vi "Lifter.vi"(1 "Joystick Speed":dbl=-0.031496062992125984) -> (0 "In Position":bool=TRUE)   [LabVIEW 2013]
uses:
  Robot Global Data.vi
  <vilib>/Rock Robotics/WPI/Joystick/WPI_JoystickGetSetRefNum.vi
panel:
  in  "Adjustment (V)":dbl
  in  "Adjust Gain (V/ms)":dbl=0.01
  in  "Limits":cluster{"Upper":dbl, "Lower":dbl}={"Upper"=3.62, "Lower"=2.5}
  out "Pot Voltage":dbl=3.41879165
  in  "Tolerance":dbl=0.01
  in  "Position Voltages":dbl[](array[numeric])=[2.5, 3.32, 3.48, 0.7, 0.7]
  in  "Motor Gain":dbl=15.0
  # "0 - Climb\n1 - Load\n2 - Pre-climb\n3 - Shoot"
  # "0 - Climb"
  # "2.5"
  # "1 - Load"
  # "3.42"
  # "3.48"
  # "2 - Pre-climb"
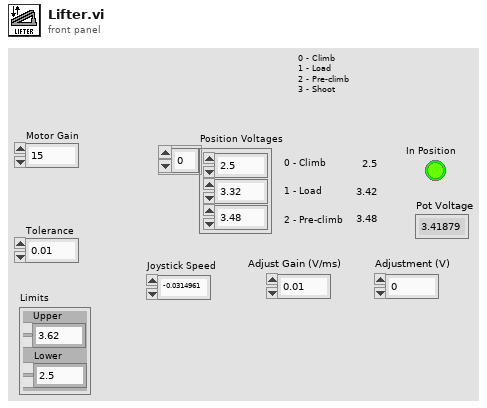
[diagram p1: front panel]
types:
  T1 = typedef "WPI_JoystickDevRef.ctl" = cluster{"Device":T2}
  T2 = typedef "WPI_JoystickDeviceEnum.ctl" = enum16{"USB 1", "USB 2", "USB 3", "USB 4", "Kinect 1", "Kinect 2"}
  T3 = typedef "WPI_AnalogChannelDevRef.ctl" = cluster{"DevStatus":errorcluster, "Analog Module":T4, "Analog Channel":T5}
  T4 = typedef "FPGA_TypedefAnalogModule.ctl" = enum16{"Analog Module 1", "Analog Module 2"}
  T5 = typedef "FPGA_AIChannel.ctl" = enum8{"AI 1", "AI 2", "AI 3", "AI 4", "AI 5", "AI 6", "AI 7", "AI 8", "Invalid"}
  T6 = typedef "WPI_JoystickButtonState.ctl" = cluster{"Button 1":bool, "Button 2":bool, "Button 3":bool, "Button 4":bool, "Button 5":bool, "Button 6":bool, "Button 7":bool, "Button 8":bool, "Button 9":bool, "Button 10":bool, "Button 11":bool, "Button 12":bool}
  T7 = typedef "WPI_MotorControlDeviceRef.ctl" = cluster{"DeviceStatus":errorcluster, "Type":enum16{"PWM", "CAN"}, "PWM":cluster{"Digital Module":T8, "PWM Channel":T9, "DeadBand":T10}, "CAN":cluster{"Device Number":u8, "Control Mode":T11, "Semaphore":T12, "Max Vout":dbl}, "Invert":bool, "TransformRef":T13, "InvTransformRef":T13}
  T8 = typedef "FPGA_TypedefDigitalModule.ctl" = enum16{"Digital Module 1", "Digital Module 2"}
  T9 = typedef "FPGA_DIOPWMChannel.ctl" = enum8{"PWM 1", "PWM 2", "PWM 3", "PWM 4", "PWM 5", "PWM 6", "PWM 7", "PWM 8", "PWM 9", "PWM 10", "Invalid"}
  T10 = typedef "WPI_PWMDeadband.ctl" = cluster{"Name":string, "maxPositivePwm":i32, "minPositivePwm":i32, "centerPwm":i32, "maxNegativePwm":i32, "minNegativePwm":i32, "angularRange":u16}
  T11 = typedef "WPI_CANJaguar_ControlMode.ctl" = enum8{"Percent VBus", "Current", "Speed", "Position", "Voltage"}
  T12 = typedef "Semaphore RefNum" = refnum<k1>
  T13 = typedef "WPI_PWMTransform_ConPane.ctl" = refnum<vi>
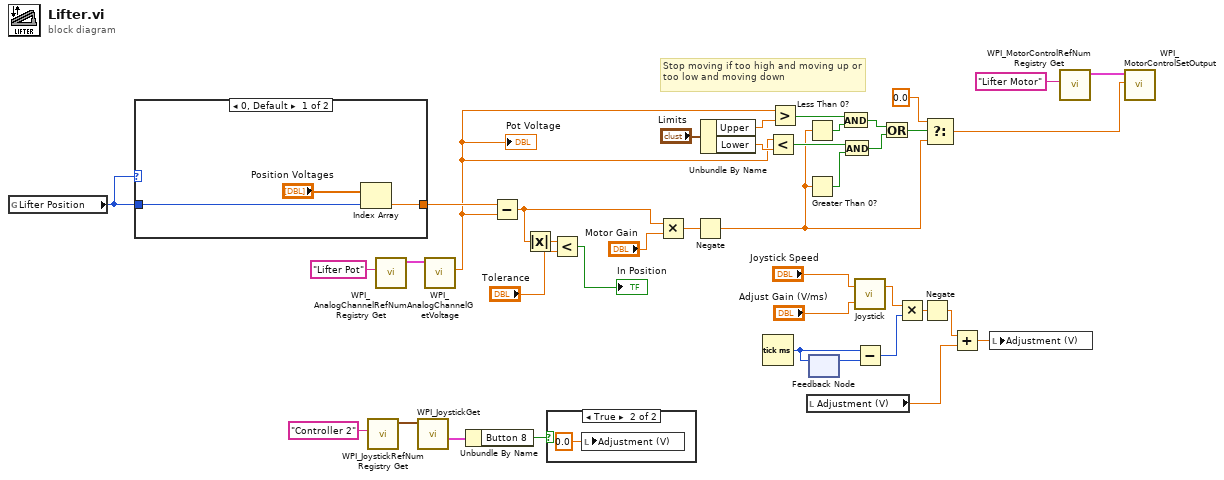
[diagram p0: block diagram]
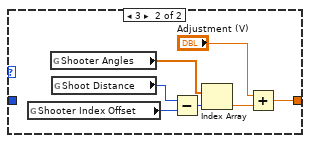
[diagram p3: hidden frame]
diagram:
  # "Stop moving if too high and moving up or too low and moving down"
  n1 = global read "Robot Global Data.vi" "Lifter Position"() -> (w30:i8)
  n2 = case shown="0, Default" w30 {
    tunnel: [w43 w45] -> w37
    tunnel: w30 -> [w42 _]
    frame 0, Default {
      n3 = Index Array(array="Position Voltages", index=w42) -> (element=w43:dbl)
    }
    frame 3 {
      n4 = global read "Robot Global Data.vi" "Shooter Index Offset"() -> (w47:i32)
      n5 = global read "Robot Global Data.vi" "Shooter Angles"() -> (w50:dbl[])
      n6 = global read "Robot Global Data.vi" "Shoot Distance"() -> (w48:i32)
      n7 = Subtract(x=w48, y=w47) -> (x-y=w49:i32)
      n8 = Index Array(array=w50, index=w49) -> (element=w46:dbl)
      n9 = Add(x="Adjustment (V)", y=w46) -> (x+y=w45:dbl)
    }
  }
  n10 = call <vilib>:"WPI_JoystickRefNum Registry Get.vi"("refnum name"="Controller 2") -> ("JoystickDevRef"=w8:T1)  [unwired: 1 in, 9 out]
  n11 = call <vilib>:"WPI_AnalogChannelRefNum Registry Get.vi"("refnum name"="Lifter Pot") -> ("AIDeviceRef"=w40:T3)  [unwired: 9 in, 1 out]
  n12 = call <vilib>:"WPI_JoystickGet.vi"("JoystickDevRef"=w8) -> ("Buttons"=w7:T6)  [unwired: 1 in, 5 out]
  n13 = call <vilib>:"WPI_AnalogChannelGetVoltage.vi"("AIDeviceRef"=w40) -> ("Voltage"=w18:dbl)  [unwired: 8 in, 2 out]
  "Pot Voltage" <- w18
  n14 = Unbundle By Name(w7) -> ("Button 8"=w6:bool)
  n15 = Subtract(x=w37, y=w18) -> (x-y=w33:dbl)
  n16 = Absolute Value(x=w33) -> (abs(x)=w32:dbl)
  n17 = case shown="True" w6 {
    frame False {
    }
    frame True {
      n18 = local write "Adjustment (V)"(0.0 ("Adjustment (V)")) -> ()
    }
  }
  n19 = Less?(x=w32, y="Tolerance") -> (x < y?=→"In Position":bool)
  n20 = Multiply(x=w33, y="Motor Gain") -> (x*y=w35:dbl)
  n21 = Negate(x=w35) -> (-x=w16:dbl)
  n22 = Unbundle By Name("Limits") -> ("Upper"=w20:dbl, "Lower"=w19:dbl)
  n23 = Tick Count (ms)() -> (millisecond timer value=w15:u32)
  n24 = Less?(x=w18, y=w19) -> (x < y?=w23:bool)
  n25 = Greater?(x=w18, y=w20) -> (0:w26:bool)
  n26 = Less Than 0?(x=w16) -> (x < 0?=w17:bool)
  n27 = Greater Than 0?(x=w16) -> (x > 0?=w22:bool)
  n28 = local read "Adjustment (V)"() -> (w2:dbl)
  n29 = feedback-in #1(w15) -> ()
  n30 = feedback #1() -> (w14:u32)  [unwired: 1 in]
  n31 = And(x=w26, y=w17) -> (x .and. y?=w25:bool)
  n32 = And(x=w23, y=w22) -> (x .and. y?=w24:bool)
  n33 = call "Joystick.vi"("Multiplier"="Adjust Gain (V/ms)", "Input"="Joystick Speed") -> ("Output"=w10:dbl)  [unwired: 1 out]
  n34 = Subtract(x=w15, y=w14) -> (x-y=w13:u32)
  n35 = Or(x=w25, y=w24) -> (x .or. y?=w27:bool)
  n36 = Multiply(x=w10, y=w13) -> (x*y=w3:dbl)
  n37 = Negate(x=w3) -> (-x=w1:dbl)
  n38 = Select(t=0.0, s=w27, f=w16) -> (s? t:f=w28:dbl)
  n39 = Add(x=w1, y=w2) -> (x+y=w4:dbl)
  n40 = local write "Adjustment (V)"(w4) -> ()
  n41 = call <vilib>:"WPI_MotorControlRefNum Registry Get.vi"("refnum name"="Lifter Motor") -> ("MotorControlDevRef"=w36:T7)  [unwired: 9 in, 1 out]
  n42 = call <vilib>:"WPI_MotorControlSetOutput.vi"("Output"=w28, "MotorControlDevRef"=w36) -> ()  [unwired: 7 in, 3 out]
